vi "Get Child Leaves by Itemlist.vi"(8 "error in":errorcluster, 10 "Item List":T1, 11 "Parent Tag":string) -> (0 "error IO":errorcluster, 3 "Children Tags":string[](array[string]))   [LabVIEW 2021]
uses:
  Control/Item List.ctl
  Control/Item Info.ctl
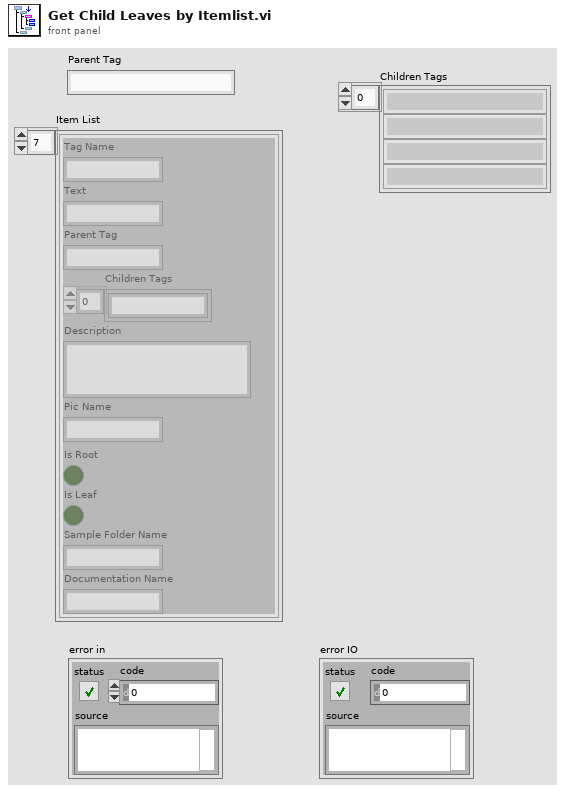
[diagram p1: front panel]
types:
  T1 = typedef "Item List.ctl" = T2[]
  T2 = typedef "Item Info.ctl" = cluster{"Tag Name":string, "Text":string, "Parent Tag":string, "Children Tags":string[], "Description":string, "Pic Name":string, "Is Root":bool, "Is Leaf":bool, "Sample Folder Name":string, "Documentation Name":string}
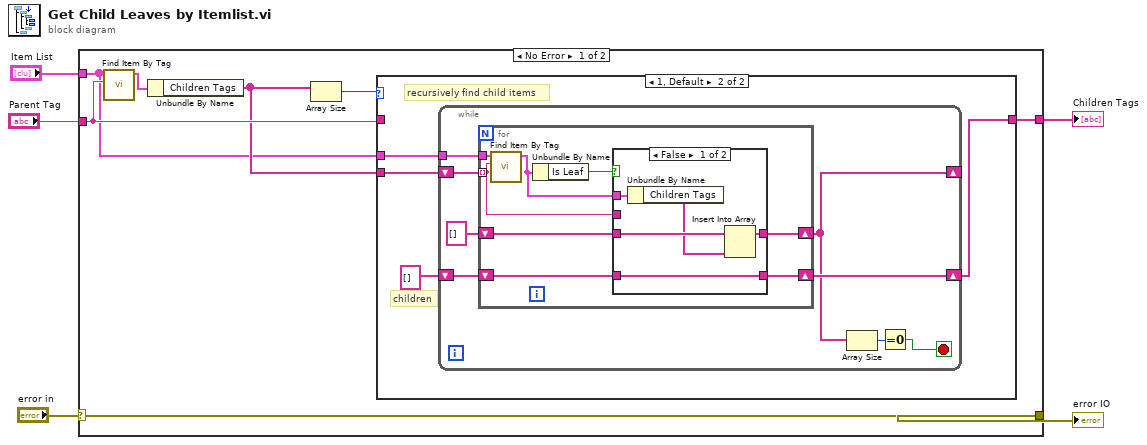
[diagram p0: block diagram]
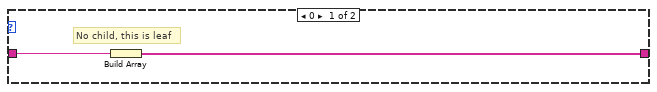
[diagram p2: hidden frame]
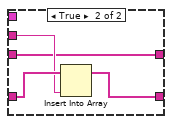
[diagram p3: hidden frame]
diagram:
  n1 = case shown="No Error" "error in" {
    selector: "error in" -> [w12 w44]
    tunnel: "Item List" -> [w7 _]
    tunnel: "Parent Tag" -> [w9 _]
    tunnel: [w12 w44] -> w2
    tunnel: [w6 _] -> w1
    frame No Error {
      n2 = call "Find Item By Tag.vi"("Tag"=w9, "Item List"=w7) -> ("Item Info"=w11:T2)  [unwired: 9 in]
      n3 = Unbundle By Name(w11) -> ("Children Tags"=w8:string[])
      n4 = Array Size(array=w8) -> (size(s)=w10:i32)
      n5 = case shown="1, Default" w10 {
        tunnel: w9 -> [w14 _]
        tunnel: [w13 w15] -> w6
        tunnel: w8 -> [_ w18]
        tunnel: w7 -> [_ w16]
        frame 0 {
          # "No child, this is leaf"
          n6 = Build Array(w14) -> (w13:string[])
        }
        frame 1, Default {
          # "recursively find child items"
          # "children"
          n7 = while {
            shift-right: [w19] -> _
            shift-left: w18 -> [w24]
            shift-right: [w21] -> w15
            shift-left: string[] [] -> [w22]
            tunnel: w16 -> [w23]
            stop <- w25 stop-if-true
            n8 = for {
              tunnel: w24 -> [w30] mode=indexing
              tunnel: w23 -> [w33]
              shift-right: [w29] -> w21
              shift-left: w22 -> [w31]
              shift-right: [w27] -> w19
              shift-left: string[] [] -> [w28]
              n9 = call "Find Item By Tag.vi"("Tag"=w30, "Item List"=w33) -> ("Item Info"=w32:T2)  [unwired: 9 in]
              n10 = Unbundle By Name(w32) -> ("Is Leaf"=w34:bool)
              n11 = case shown="False" w34 {
                tunnel: w32 -> [w39 _]
                tunnel: w31 -> [w38 w43]
                tunnel: w30 -> [_ w42]
                tunnel: [w38 w41] -> w29
                tunnel: w28 -> [w37 w40]
                tunnel: [w35 w40] -> w27
                frame False {
                  n12 = Unbundle By Name(w39) -> ("Children Tags"=w36:string[])
                  n13 = Insert Into Array(array=w37, new element=w36) -> (w35:string[])  [unwired: 1 in]
                }
                frame True {
                  n14 = Insert Into Array(array=w43, new element=w42) -> (w41:string[])  [unwired: 1 in]
                }
              }
            }
            n15 = Array Size(array=w19) -> (size(s)=w26:i32)
            n16 = Equal To 0?(x=w26) -> (x = 0?=w25:bool)
          }
        }
      }
    }
    frame Error {
    }
  }
  "Children Tags" <- w1
  "error IO" <- w2
